vi "Simple H5Awrite (Variant).vi"(4 "Value":variant, 5 "operation (open or create)":T1=enum."create or replace", 6 "error in (no error)":errorcluster, 8 "Name":string, 9 "HDF5 Ref":T2) -> (0 "error out":errorcluster, 3 "HDF5 Ref out":T2)   [LabVIEW 2017]
doc: "Writes data to an attribute."
uses:
  <vilib>/UPVI/lvhdf5/library.llb/HDF5 Ref.ctl
  <vilib>/UPVI/lvhdf5/attribute.llb/LVH5A Operation.ctl
panel:
  # "LVHDF5 Toolkit\nCopyright (c) 2005-2013 by Jason D. Sommerville\nCopyright (c) 2014 by UPVI, LLC.\n\nThis use and distribution of this file is governed by the terms found in \nLICENSE.txt distributed with this toolkit and installed at\n <user.lib>\\_lvhdf5\\LICENSE.txt"
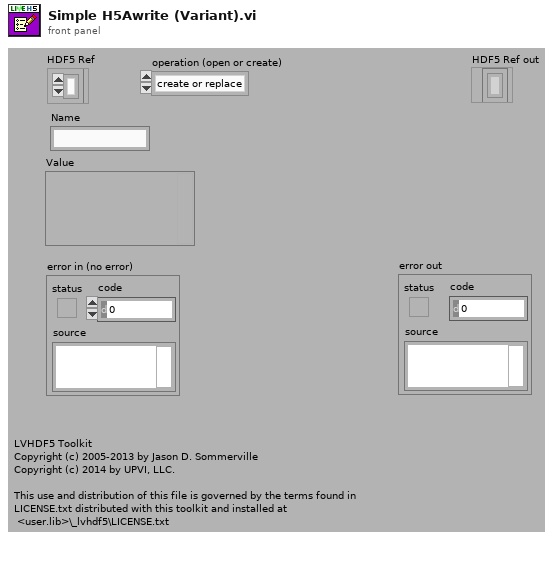
[diagram p1: front panel]
types:
  T1 = typedef "LVH5A Operation.ctl" = enum16{"open", "replace", "create", "open or create", "create or replace", "create or replace with confirmation"}
  T2 = typedef "HDF5 Ref.ctl" = refnum<k1>
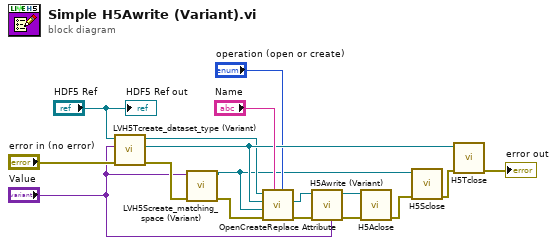
[diagram p0: block diagram]
diagram:
  n1 = call <vilib>:"LVH5Tcreate_dataset_type (Variant).vi"("error in (no error)"="error in (no error)", "Data"="Value", "HDF5 Ref"="HDF5 Ref") -> ("error out"=w4:errorcluster, "HDF5 Type Ref"=w9:T2, "HDF5 Ref out"=w8:T2)  [unwired: 4 in, 2 out]
  n2 = call <vilib>:"LVH5Screate_matching_space (Variant).vi"("error in (no error)"=w4, "Data"="Value") -> ("error out"=w3:errorcluster, "HDF5 Dataspace Ref"=w2:T2)  [unwired: 6 in]
  n3 = call <vilib>:"OpenCreateReplace Attribute.vi"("operation (open or create)"="operation (open or create)", "Name"="Name", "error in (no error)"=w3, "HDF5 Dataspace Ref"=w2, "HDF5 Datatype Ref"=w9, "HDF5 Ref"=w8) -> ("error out"=w11:errorcluster, "HDF5 Attr Ref"=w6:T2)  [unwired: 3 in, 1 out]
  n4 = call <vilib>:"H5Awrite (Variant).vi"("Data"="Value", "error in (no error)"=w11, "HDF5 Attr Ref"=w6) -> ("error out"=w12:errorcluster, "HDF5 Attr Ref out"=w13:T2)  [unwired: 5 in]
  n5 = call <vilib>:"H5Aclose.vi"("error in (no error)"=w12, "HDF5 Dataset Ref"=w13) -> ("error out"=w14:errorcluster)  [unwired: 7 in]
  n6 = call <vilib>:"H5Sclose.vi"("error in (no error)"=w14, "HDF5 Dataspace Ref"=w2) -> ("error out"=w15:errorcluster)  [unwired: 7 in]
  n7 = call <vilib>:"H5Tclose.vi"("error in (no error)"=w15, "HDF5 Datatype Ref"=w9) -> ("error out"=→"error out":errorcluster)  [unwired: 7 in]
  "HDF5 Ref out" <- "HDF5 Ref"
